vi "HEALTH_LABVIEW_V2.vi"() -> ()   [LabVIEW 2026]
panel:
  out "Waveform Chart":dbl(graph)
  out "HEATER POWER OUTPUT":dbl(knob) scale=0.0..100.0
  in  "TARGET HEATER TEMP (C)":dbl
  in  "HEATER ON/OFF":bool
  out "HEATER TEMP (C)":dbl(knob) scale=20.0..90.0
  out "HEATER TEMP (C)":dbl format="%.2f"
  in  "stop":bool
  out "Error String":string
  out "error out":errorcluster
  out "ConnectionType Out":i32
  out "DeviceType Out":i32
  in  "Identifier":string="LJM_idANY"
  in  "ConnectionType":string="LJM_ctANY"
  in  "DeviceType":string="LJM_dtANY"
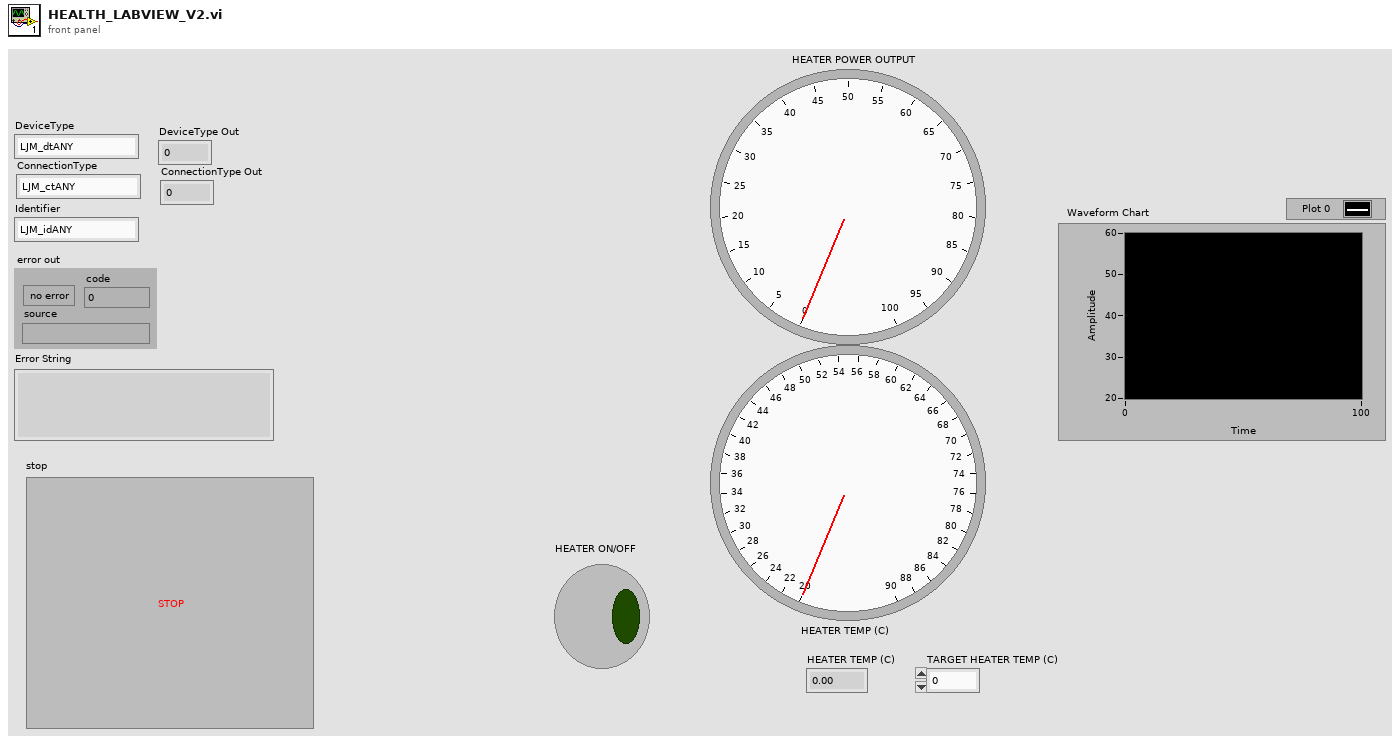
[diagram p1: front panel]
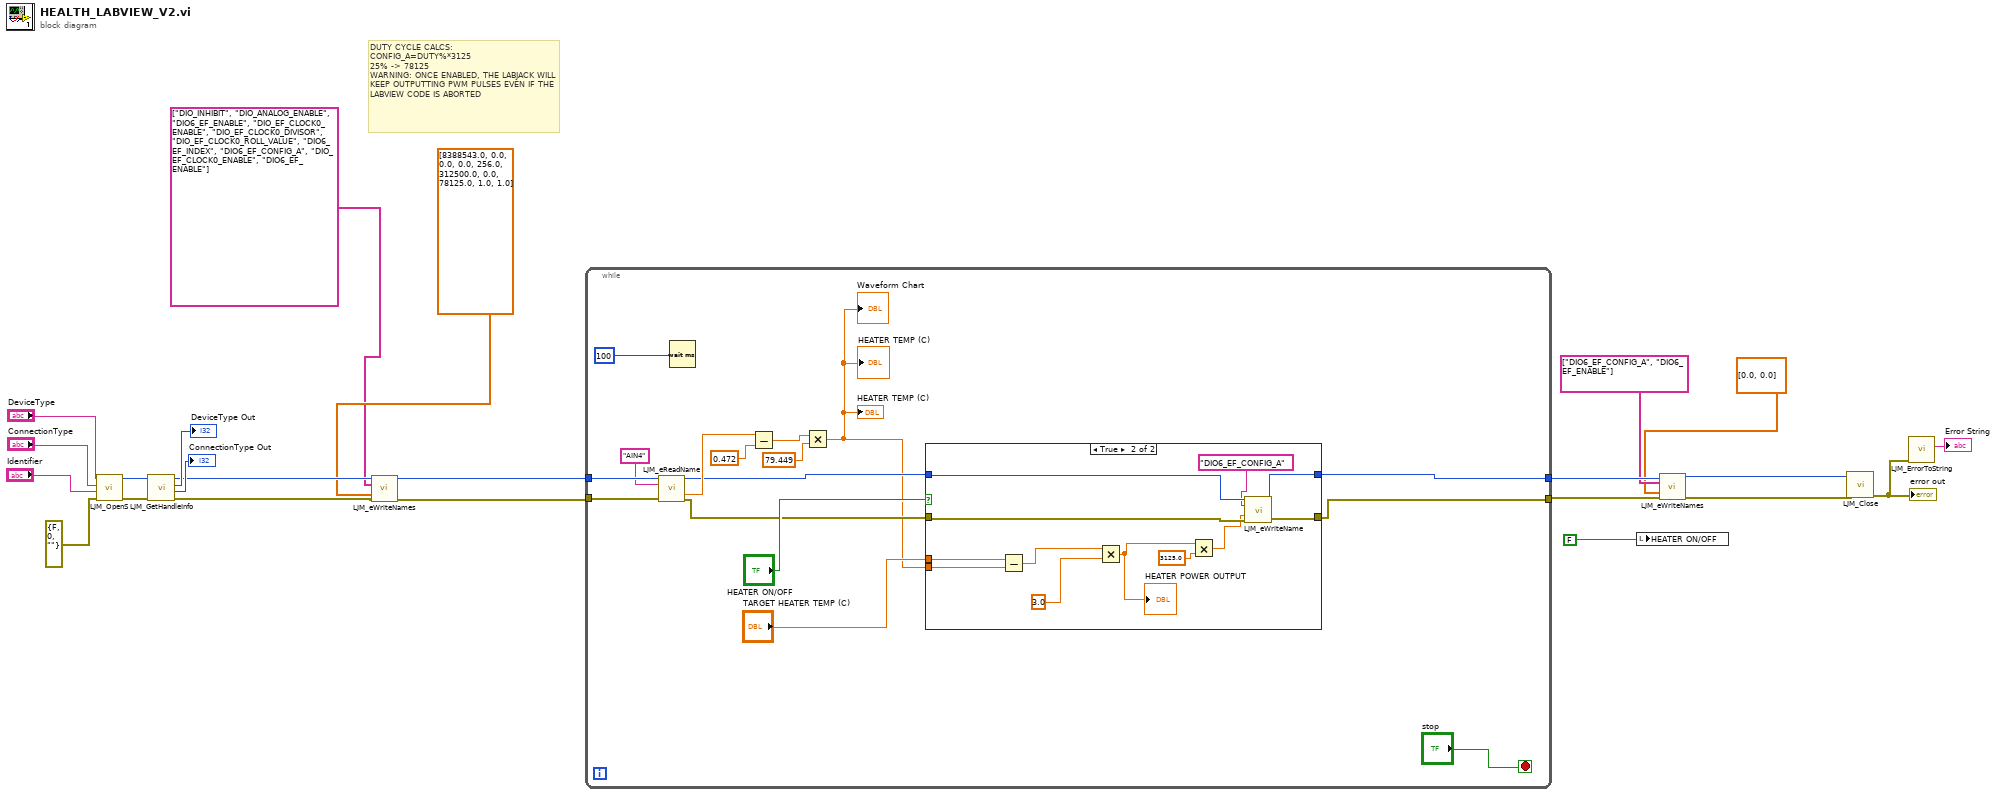
[diagram p0: block diagram]
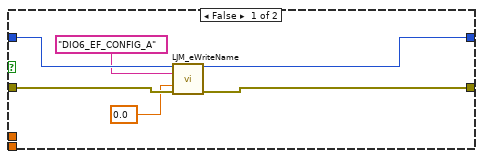
[diagram p2: hidden frame]
diagram:
  # "DUTY CYCLE CALCS:\nCONFIG_A=DUTY%*3125\n25% -> 78125\nWARNING: ONCE ENABLED, THE LABJACK WILL KEEP OUTPUTTING PWM PULSES EVEN IF THE LABVIEW CODE IS ABORTED"
  n1 = call "LJM_OpenS.vi"("error in"=errorcluster {"status"=FALSE, "code"=0, "source"=""} ("error in (no error)"), "Identifier"="Identifier", "ConnectionType"="ConnectionType", "DeviceType"="DeviceType") -> ("error out"=w22:errorcluster, "Handle"=w21:i32)  [unwired: 6 in]
  n2 = call "LJM_GetHandleInfo.vi"("error in"=w22, "Handle In"=w21) -> ("error out"=w12:errorcluster, "ConnectionType"=→"ConnectionType Out":i32, "DeviceType"=→"DeviceType Out":i32, "Handle Out"=w13:i32)  [unwired: 2 in, 4 out]
  n3 = call "LJM_eWriteNames.vi"("Handle In"=w13, "aNames"=string[] ["DIO_INHIBIT", "DIO_ANALOG_ENABLE", "DIO6_EF_ENABLE", "DIO_EF_CLOCK0_ENABLE", "DIO_EF_CLOCK0_DIVISOR", "DIO_EF_CLOCK0_ROLL_VALUE", "DIO6_EF_INDEX", "DIO6_EF_CONFIG_A", "DIO_EF_CLOCK0_ENABLE", "DIO6_EF_ENABLE"], "aValuesIn"=dbl[] [8388543.0, 0.0, 0.0, 0.0, 256.0, 312500.0, 0.0, 78125.0, 1.0, 1.0], "error in"=w12) -> ("Handle Out"=w10:i32, "error out"=w11:errorcluster)  [unwired: 9 in, 1 out]
  n4 = while {
    tunnel: w11 -> [w33]
    tunnel: w10 -> [w34]
    tunnel: [w27] -> w7
    tunnel: [w28] -> w6
    stop <- "stop" stop-if-true
    n5 = call "LJM_eReadName.vi"("Handle In"=w34, "Name"="AIN4", "error in"=w33) -> ("Handle Out"=w30:i32, "Value"=w35:dbl, "error out"=w29:errorcluster)  [unwired: 10 in]
    n6 = Wait (ms)(milliseconds to wait=u32 100) -> ()  [unwired: 1 out]
    n7 = Subtract(x=w35, y=0.472 ("Address 2")) -> (x-y=w38:dbl)
    n8 = Multiply(x=w38, y=79.449 ("Address 2")) -> (x*y=w24:dbl)
    "HEATER TEMP (C)" <- w24
    "HEATER TEMP (C)" <- w24
    "Waveform Chart" <- w24
    n9 = case shown="True" "HEATER ON/OFF" {
      tunnel: w30 -> [w42 w57]
      tunnel: w29 -> [w43 w56]
      tunnel: [w44 w55] -> w28
      tunnel: [w45 w54] -> w27
      tunnel: "TARGET HEATER TEMP (C)" -> [_ w50]
      tunnel: w24 -> [_ w49]
      frame False {
        n10 = call "LJM_eWriteName.vi"("Handle In"=w42, "Name"="DIO6_EF_CONFIG_A", "Value"=0.0, "error in"=w43) -> ("Handle Out"=w45:i32, "error out"=w44:errorcluster)  [unwired: 10 in]
      }
      frame True {
        n11 = Subtract(x=w50, y=w49) -> (x-y=w47:dbl)
        n12 = Multiply(x=w47, y=3.0 ("PROPORTIONAL GAIN")) -> (x*y=w46:dbl)
        "HEATER POWER OUTPUT" <- w46
        n13 = Multiply(x=w46, y=3125.0) -> (x*y=w52:dbl)
        n14 = call "LJM_eWriteName.vi"("Handle In"=w57, "Name"="DIO6_EF_CONFIG_A", "Value"=w52, "error in"=w56) -> ("Handle Out"=w54:i32, "error out"=w55:errorcluster)  [unwired: 10 in]
      }
    }
  }
  n15 = local write "HEATER ON/OFF"(FALSE ("HEATER ON/OFF 2")) -> ()
  n16 = call "LJM_eWriteNames.vi"("Handle In"=w7, "aNames"=string[] ["DIO6_EF_CONFIG_A", "DIO6_EF_ENABLE"], "aValuesIn"=dbl[] [0.0, 0.0], "error in"=w6) -> ("Handle Out"=w4:i32, "error out"=w5:errorcluster)  [unwired: 9 in, 1 out]
  n17 = call "LJM_Close.vi"("error in"=w5, "Handle"=w4) -> ("error out"=w14:errorcluster)  [unwired: 9 in]
  "error out" <- w14
  n18 = call "LJM_ErrorToString.vi"("error in"=w14) -> ("String"=→"Error String":string)  [unwired: 10 in]
